vi "Unpack Value Change.vi"(11 "ValueChangeMsg":refnum<class "ValueChangeMsg.lvclass">) -> (0 "New Value":variant, 1 "Time":u32, 2 "Control Label":string, 3 "Ctl Refnum":refnum<vi>, 4 "Old Value":variant)   [LabVIEW 2020, in "MVA Framework.lvlib" / "ActorEvents.lvlib" / "ValueChangeMsg.lvclass"]
doc: "<License>\nCopyright © 2017 Composed Systems, LLC | All rights reserved\nwww.composed.io\n\nAuthor: Ethan Stern <ethan.stern@composed.io>\n\nThis software is provided \"AS IS\" WITHOUT WARRANTIES, either express or implied, AND IS FOR EDUCATIONAL PURPOSES ONLY.\n</License>"
uses:
  ValueChangeMsg.lvclass
  ValueChangeMsg.lvclass/ValueChangeMsg.ctl
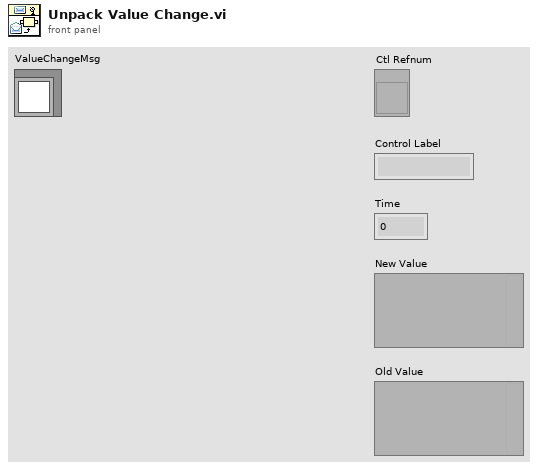
[diagram p1: front panel]
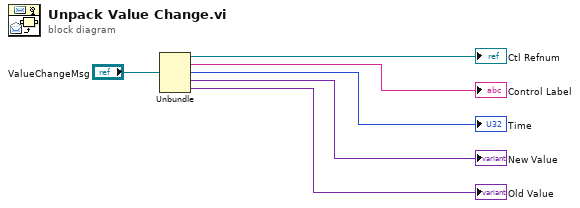
[diagram p0: block diagram]
diagram:
  n1 = Unbundle("ValueChangeMsg") -> (→"Ctl Refnum":refnum<vi>, →"Control Label":string, →"Time":u32, →"New Value":variant, →"Old Value":variant)
